vi "Open and Save All Library VIs.vi"(8 "error in (no error)":errorcluster, 11 "library ref":refnum<vi>) -> (0 "error out":errorcluster)   [LabVIEW 2017, in "Build Automation.lvlib"]
uses:
  Build Automation.lvlib
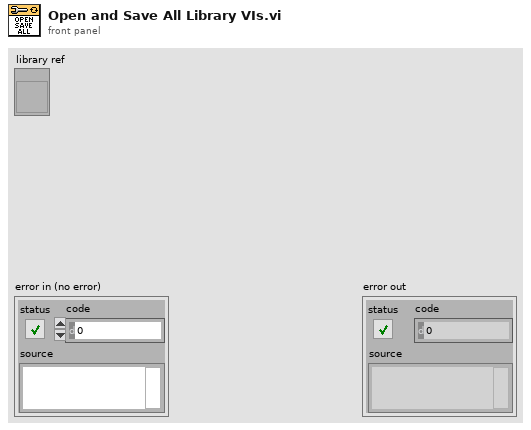
[diagram p1: front panel]
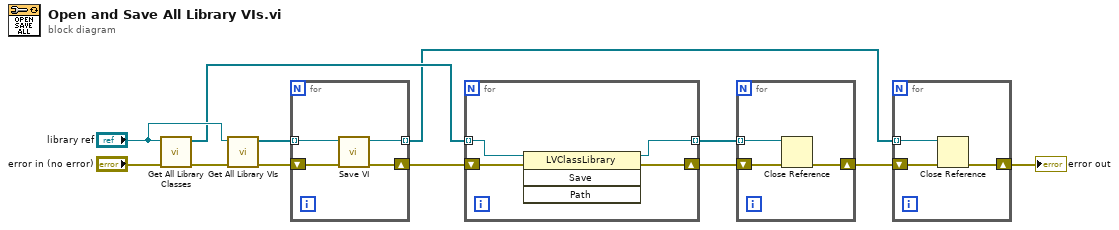
[diagram p0: block diagram]
diagram:
  n1 = call "Get All Library Classes.vi"("error in (no error)"="error in (no error)", "library ref"="library ref") -> ("error out"=w11:errorcluster, "class refs"=w6:refnum<vi>[])  [unwired: 8 in]
  n2 = call "Get All Library VIs.vi"("error in (no error)"=w11, "library ref"="library ref") -> ("error out"=w9:errorcluster, "vi refs"=w8:refnum<vi>[])  [unwired: 8 in]
  n3 = for {
    shift-right: [w14] -> w7
    shift-left: w9 -> [w16]
    tunnel: w8 -> [w15] mode=indexing
    tunnel: [w13] -> w2 mode=indexing
    n4 = call "Save VI.vi"("error in (no error)"=w16, "vi ref in"=w15) -> ("error out"=w14:errorcluster, "vi ref out"=w13:refnum<vi>)  [unwired: 8 in]
  }
  n5 = for {
    shift-right: [w19] -> w5
    shift-left: w7 -> [w20]
    tunnel: w6 -> [w18] mode=indexing
    tunnel: [w17] -> w4 mode=indexing
    n6 = invoke class="LVClassLibrary" method="Save"(reference=w18, error in=w20) -> (reference out=w17:refnum<vi>, error out=w19:errorcluster)  [unwired: 2 in, 2 out]
  }
  n7 = for {
    shift-right: [w21] -> w3
    shift-left: w5 -> [w23]
    tunnel: w4 -> [w22] mode=indexing
    n8 = Close Reference(reference=w22, error in (no error)=w23) -> (error out=w21:errorcluster)
  }
  n9 = for {
    shift-right: [w24] -> w1
    shift-left: w3 -> [w26]
    tunnel: w2 -> [w25] mode=indexing
    n10 = Close Reference(reference=w25, error in (no error)=w26) -> (error out=w24:errorcluster)
  }
  "error out" <- w1
